vi "AndorReturn2Error.vi"(8 "error in (no error)":errorcluster, 11 "Camera return":u32) -> (0 "error out":errorcluster)   [LabVIEW 2018, in "AndorOWN.lvlib"]
uses:
  AndorOWN.lvlib
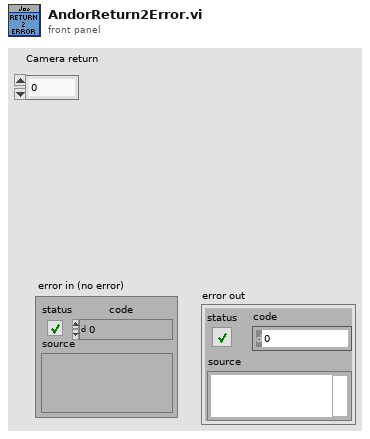
[diagram p1: front panel]
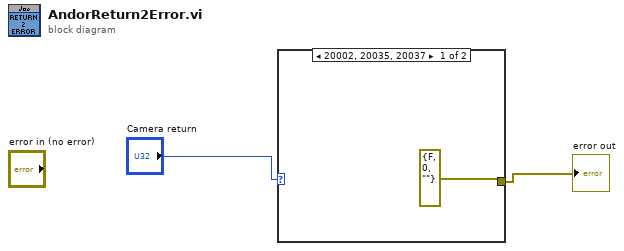
[diagram p0: block diagram]
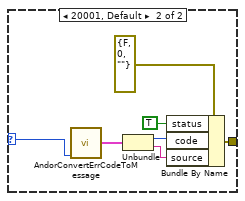
[diagram p2: hidden frame]
diagram:
  n1 = case shown="20002, 20035, 20037" "Camera return" {
    selector: "Camera return" -> [_ w4]
    tunnel: [errorcluster {"status"=FALSE, "code"=0, "source"=""} ("error constant") w6] -> w2
    frame 20002, 20035, 20037 {
    }
    frame 20001, Default {
      n2 = call "AndorConvertErrCodeToMessage.vi"("function return"=w4) -> ("Element Return"=w10:cluster{i32, string})  [unwired: 10 in]
      n3 = Unbundle(w10) -> (w8:i32, w9:string)
      n4 = Bundle By Name(cluster=errorcluster {"status"=FALSE, "code"=0, "source"=""} ("error constant"), "status"=TRUE, "code"=w8, "source"=w9) -> (w6:errorcluster)
    }
  }
  "error out" <- w2
